vi "Untitled 2.vi"() -> ()   [LabVIEW 2014]
panel:
  out "Waveform Chart":dynamicdata(graph)
  in  "stop":bool
  in  "Slide 2":dbl(slide) scale=0.0..200.0
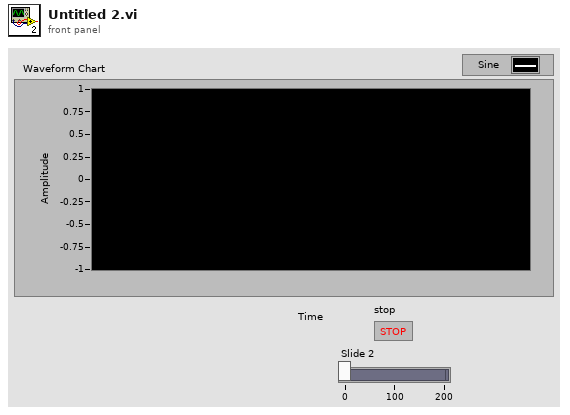
[diagram p1: front panel]
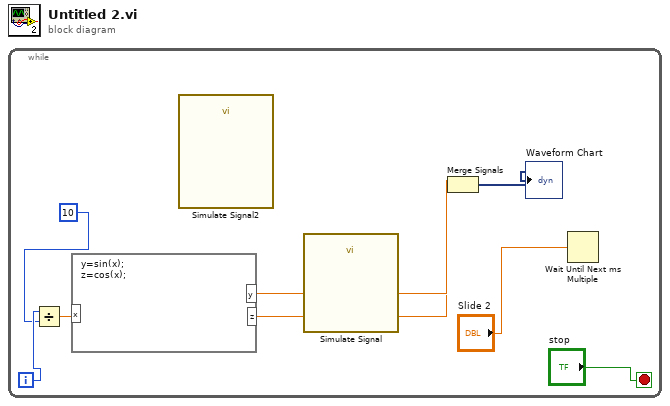
[diagram p0: block diagram]
diagram:
  n1 = while {
    i -> [w2]
    stop <- "stop" stop-if-true
    n2 = Divide(x=w2, y=10) -> (x/y=w3:dbl)
    n3 = formula code="y=sin(x);\nz=cos(x);"("x"=w3) -> ("z"=w4:dbl, "y"=w5:dbl)
    n4 = call "Simulate Signal2"() -> ()  [unwired: 14 in, 2 out]
    n5 = call "Simulate Signal"() -> ()  [unwired: 14 in, 2 out]
    n6 = Merge Signals(w5, w4) -> (→"Waveform Chart":dynamicdata)
    n7 = Wait Until Next ms Multiple(millisecond multiple="Slide 2") -> ()  [unwired: 1 out]
  }
